vi "LoadConfiguration.vi"(0 "instruction target in":refnum<class "niInstr Instruction Target v1 Host.lvclass">, 1 "Configuration":T1 {"dT" format="%#_13g"; "ClkRate" format="%#_13g"}, 5 "QuadEncContext in":refnum<class "niInstr Instruction Framework Context v1 Host.lvclass">, 11 "error in (no error)":errorcluster) -> (4 "instruction target out":refnum<class "niInstr Instruction Target v1 Host.lvclass">, 6 "QuadEncContext out":refnum<class "niInstr Instruction Framework Context v1 Host.lvclass">, 15 "error out":errorcluster)   [LabVIEW 2015, in "QuadEncInterface.lvlib"]
uses:
  QuadEncInterface.lvlib
  <instrlib>/_niInstr/Instruction Framework/v1/Host/Instruction Framework Context/niInstr Instruction Framework Context v1 Host.lvclass
  <instrlib>/_niInstr/Instruction Framework/v1/Host/Instruction Target/niInstr Instruction Target v1 Host.lvclass
  Configuration.ctl
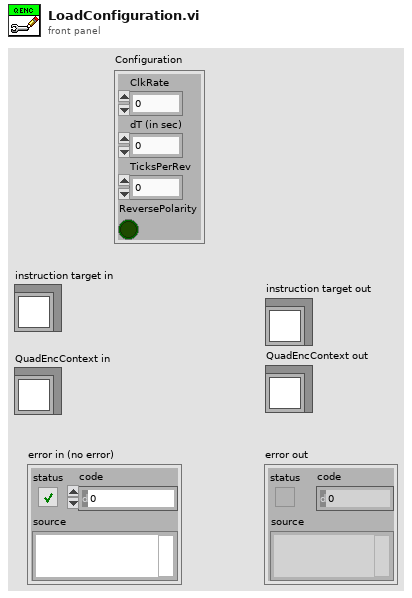
[diagram p1: front panel]
types:
  T1 = typedef "QuadEncInterface.lvlib/Configuration.ctl" = cluster{"ClkRate":dbl, "dT":dbl, "TicksPerRev":u32, "ReversePolarity":bool}
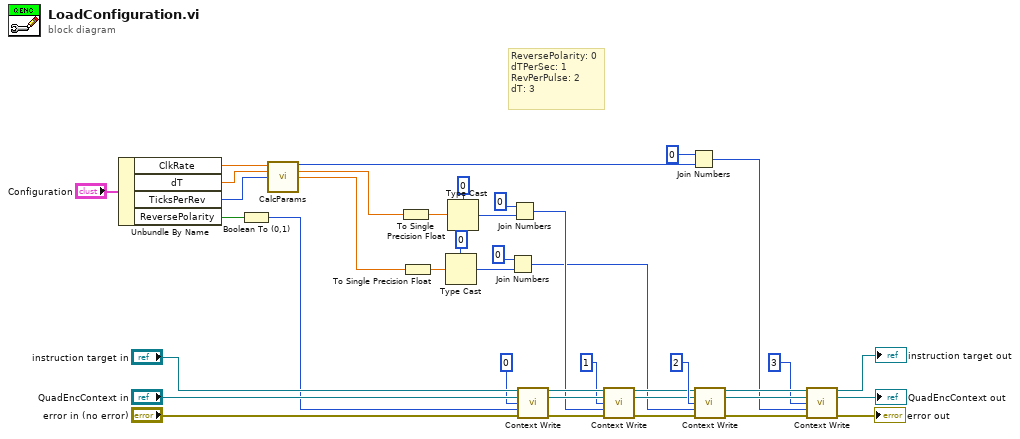
[diagram p0: block diagram]
diagram:
  # "ReversePolarity: 0\ndTPerSec: 1\nRevPerPulse: 2\ndT: 3"
  n1 = Unbundle By Name("Configuration") -> ("ClkRate"=w22:dbl, "dT"=w19:dbl, "TicksPerRev"=w18:u32, "ReversePolarity"=w21:bool)
  n2 = Boolean To (0,1)(Boolean=w21) -> (0, 1=w20:i16)
  n3 = call "CalcParams.vi"("ClkRate"=w22, "dT"=w19, "TicksPerRev"=w18) -> ("dT"=w17:u32, "dTPerSec"=w3:dbl, "RevPerPulse"=w1:dbl)  [unwired: 10 in]
  n4 = To Single Precision Float(number=w3) -> (single precision float=w4:sgl)
  n5 = To Single Precision Float(number=w1) -> (single precision float=w2:sgl)
  n6 = Type Cast(type=u32 0, x=w2) -> (*(type *) &x=w9:u32)
  n7 = Type Cast(type=u32 0, x=w4) -> (*(type *) &x=w11:u32)
  n8 = Join Numbers(hi=u32 0, lo=w9) -> ((hi.lo)=w7:u64)
  n9 = Join Numbers(hi=u32 0, lo=w11) -> ((hi.lo)=w8:u64)
  n10 = call <instrlib>:"Context Write.vi"("instruction target in"="instruction target in", "context in"="QuadEncContext in", "address"=u64 0, "data"=w20, "error in"="error in (no error)") -> ("instruction target out"=w31:refnum<class "niInstr Instruction Target v1 Host.lvclass">, "context out"=w28:refnum<class "niInstr Instruction Framework Context v1 Host.lvclass">, "error out"=w27:errorcluster)  [unwired: 8 in]
  n11 = call <instrlib>:"Context Write.vi"("instruction target in"=w31, "context in"=w28, "address"=u64 1, "data"=w8, "error in"=w27) -> ("instruction target out"=w30:refnum<class "niInstr Instruction Target v1 Host.lvclass">, "context out"=w29:refnum<class "niInstr Instruction Framework Context v1 Host.lvclass">, "error out"=w26:errorcluster)  [unwired: 8 in]
  n12 = Join Numbers(hi=u32 0, lo=w17) -> ((hi.lo)=w15:u64)
  n13 = call <instrlib>:"Context Write.vi"("instruction target in"=w30, "context in"=w29, "address"=u64 2, "data"=w7, "error in"=w26) -> ("instruction target out"=w37:refnum<class "niInstr Instruction Target v1 Host.lvclass">, "context out"=w36:refnum<class "niInstr Instruction Framework Context v1 Host.lvclass">, "error out"=w35:errorcluster)  [unwired: 8 in]
  n14 = call <instrlib>:"Context Write.vi"("instruction target in"=w37, "context in"=w36, "address"=u64 3, "data"=w15, "error in"=w35) -> ("instruction target out"=→"instruction target out":refnum<class "niInstr Instruction Target v1 Host.lvclass">, "context out"=→"QuadEncContext out":refnum<class "niInstr Instruction Framework Context v1 Host.lvclass">, "error out"=→"error out":errorcluster)  [unwired: 8 in]
